vi "Disable Lockstep.vi"(8 "error in (no error)":errorcluster, 9 "Device Number":string, 10 "Lockstep Group (1)":u8=1, 11 "VISA resource name":refnum<visa-resource-name>) -> (0 "error out":errorcluster, 3 "VISA resource name out":refnum<visa-resource-name>)   [LabVIEW 2013, in "Zaber A Series.lvlib"]
doc: "Disables a lockstep group that was previously enabled using the Enable Lockstep VI. After this, the axes that were part of the group will be able to move independently using the normal move commands.\n\nThis VI does not check in advance for error conditions such as lockstep not being supported on the device or the group number not having been enabled previously.\n\nThis VI requires that the Initialize VI has been called with the same serial port."
uses:
  Zaber A Series.lvlib
  Private/All Commands.ctl
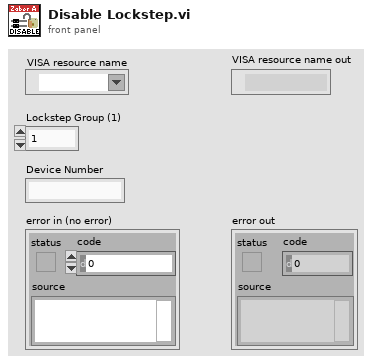
[diagram p1: front panel]
types:
  T1 = typedef "Zaber A Series.lvlib/All Commands.ctl" = string
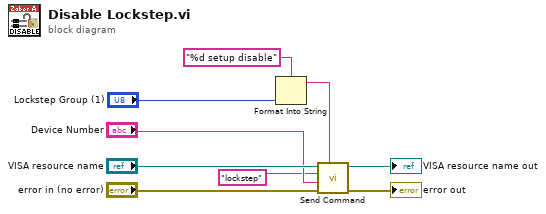
[diagram p0: block diagram]
diagram:
  n1 = Format Into String(format string="%d setup disable", "Lockstep Group (1)") -> (resulting string=w2:string)  [unwired: 2 in, 1 out]
  n2 = call "Send Command.vi"("Data"=w2, "error in (no error)"="error in (no error)", "Device and Axis"="Device Number", "Command"=T1 "lockstep" ("Complete Command List"), "VISA resource name"="VISA resource name") -> ("error out"=→"error out":errorcluster, "VISA resource name out"=→"VISA resource name out":refnum<visa-resource-name>)  [unwired: 1 in, 4 out]
